vi "processData.vi"(8 "error in (no error)":errorcluster, 10 "model":refnum<class "Model.lvclass">, 11 "WaitingForSettledSTState in":refnum<class "WaitingForSettledSTState.lvclass">) -> (0 "error out":errorcluster, 2 "model 2":refnum<class "Model.lvclass">, 3 "WaitingForSettledSTState out":refnum<class "WaitingForSettledSTState.lvclass">)   [LabVIEW 2015, in "WaitingForSettledSTState.lvclass"]
uses:
  WaitingForSettledSTState.lvclass
  Model/Model/Model.lvclass
  TestingStiffnessState/TestingStiffnessState.lvclass
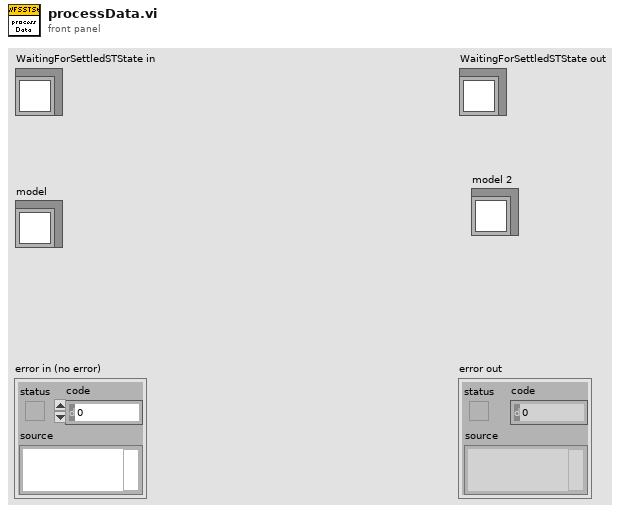
[diagram p1: front panel]
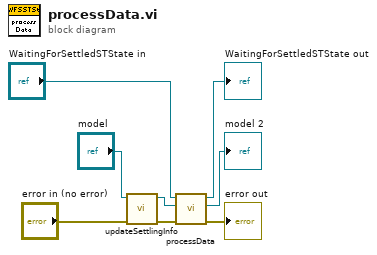
[diagram p0: block diagram]
diagram:
  n1 = call "updateSettlingInfo.vi"("error in (no error)"="error in (no error)", "Model in"="model") -> ("error out"=w2:errorcluster, "Model out"=w4:refnum<class "Model.lvclass">)  [unwired: 8 in]
  n2 = call-parent "processData.vi"("error in (no error)"=w2, "model"=w4, "TestingState in"="WaitingForSettledSTState in") -> ("error out"=→"error out":errorcluster, "model 2"=→"model 2":refnum<class "Model.lvclass">, "TestingState out"=→"WaitingForSettledSTState out":refnum<class "WaitingForSettledSTState.lvclass">)  [unwired: 6 in]
